vi "Read eventEvents.vi"(8 "error in (no error)":errorcluster, 11 "SAL_Events in":refnum<class "SAL_Events.lvclass">) -> (0 "error out":errorcluster, 2 "eventEvents":T1, 3 "SAL_Events out":refnum<class "SAL_Events.lvclass">)   [LabVIEW 2016, in "SAL_Events.lvclass"]
uses:
  SAL_Events.lvclass
  typedefs/eventsEvents.ctl
  SALLV_dome/DataTypes/logevent_AppliedSettingsMatchStart.ctl
  SALLV_dome/DataTypes/logevent_ErrorCode.ctl
  SALLV_dome/DataTypes/logevent_SettingVersions.ctl
  SALLV_dome/DataTypes/logevent_StateChanged.ctl
  SALLV_dome/DataTypes/logevent_SummaryState.ctl
  SAL_Events.lvclass/SAL_Events.ctl
  SALLV_dome/SALLV_dome.lvlib
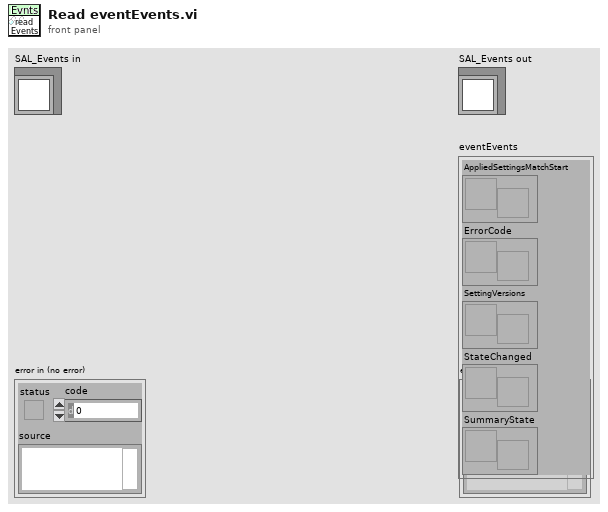
[diagram p1: front panel]
types:
  T1 = typedef "eventsEvents.ctl" = cluster{"AppliedSettingsMatchStart":refnum<user-event>, "ErrorCode":refnum<user-event>, "SettingVersions":refnum<user-event>, "StateChanged":refnum<user-event>, "SummaryState":refnum<user-event>}
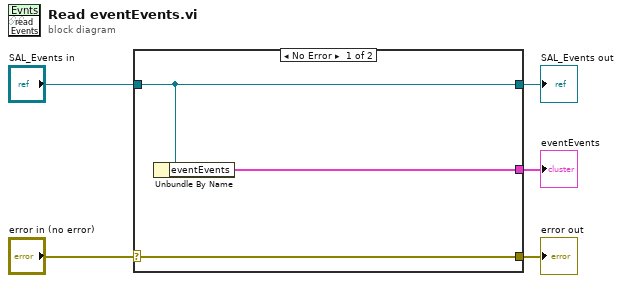
[diagram p0: block diagram]
diagram:
  n1 = case shown="No Error" "error in (no error)" {
    selector: "error in (no error)" -> [w8 w9]
    tunnel: [w8 w9] -> w4
    tunnel: [w7 w10] -> w2
    tunnel: "SAL_Events in" -> [w7 w10]
    tunnel: [w6 _] -> w1
    frame No Error {
      n2 = Unbundle By Name(w7) -> ("eventEvents"=w6:T1)
    }
    frame Error {
    }
  }
  "error out" <- w4
  "SAL_Events out" <- w2
  "eventEvents" <- w1
